vi "B sweep PL.vi"() -> ()   [LabVIEW 2012]
uses:
  <vilib>/Analysis/1siggen.llb/Ramp Pattern by Samples.vi
  <vilib>/Utility/file.llb/Write To Spreadsheet File (DBL).vi
  <vilib>/Analysis/NI_AALBase.lvlib
panel:
  in  "Y Parameters":T1={"Number of Y Steps"=200, "Max Y (V)"=2.0, "Min Y (V)"=-2.0}
  in  "X":T2={"Number of X Steps"=200, "Max X (V)"=2.0, "Min X (V)"=-2.0}
  out "Numeric":dbl
  out "Average intensity (cts/s)":dbl
  in  "file path (dialog if empty)":path
  in  "Time Target (s)":dbl=10.0
  in  "Z Position":dbl
  in  "Y Position":dbl
  in  "X Position":dbl
  in  "Z-track?":bool
  in  "start":dbl format="%0.2f"
  in  "end":dbl=1.0 format="%0.2f"
  in  "samples":i32=128
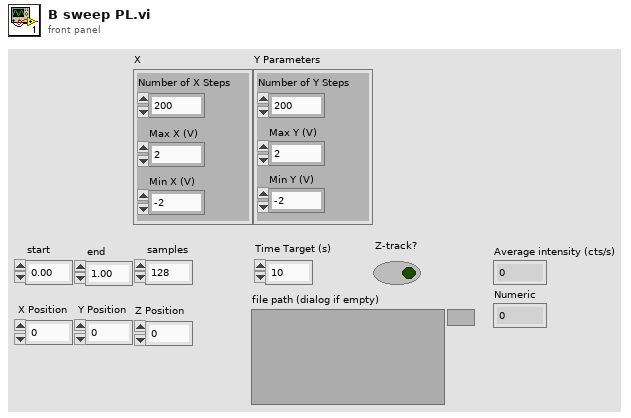
[diagram p1: front panel]
types:
  T1 = cluster{"Number of Y Steps":i32, "Max Y (V)":dbl, "Min Y (V)":dbl}
  T2 = cluster{"Number of X Steps":i32, "Max X (V)":dbl, "Min X (V)":dbl}
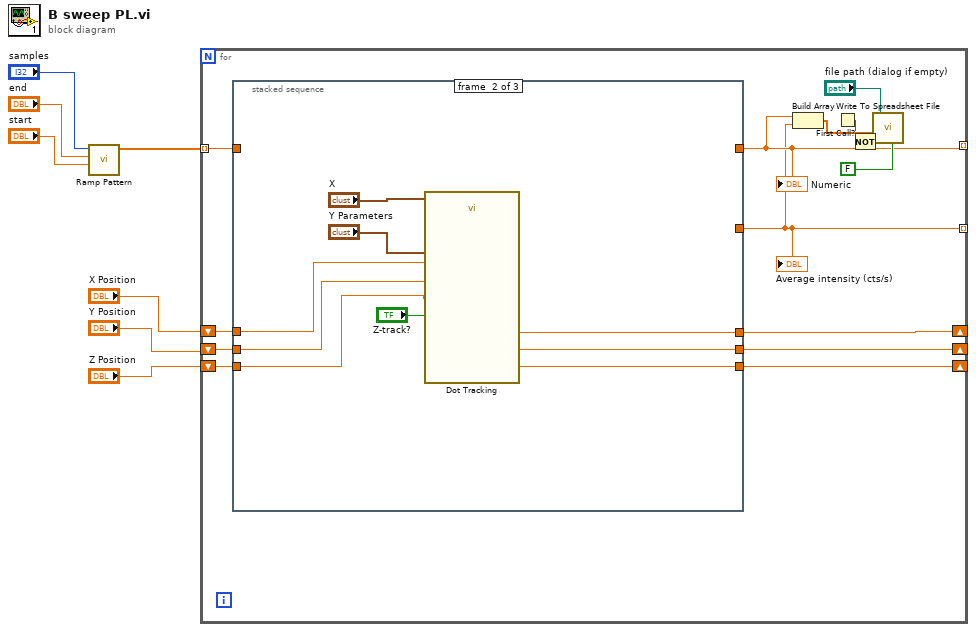
[diagram p0: block diagram]
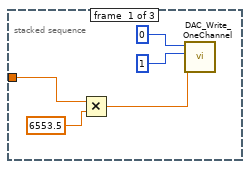
[diagram p2: hidden frame]
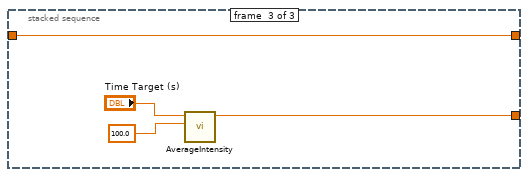
[diagram p3: hidden frame]
diagram:
  n1 = call-poly <vilib>:"Ramp Pattern.vi"("start"="start", "end"="end", "samples"="samples") -> ("Ramp Pattern"=w4:dbl[])  [unwired: 7 in, 1 out]
  n2 = for {
    tunnel: w4 -> [w21] mode=indexing
    shift-right: [w18] -> _
    shift-left: "Z Position" -> [w15]
    shift-right: [w19] -> _
    shift-left: "Y Position" -> [w16]
    shift-right: [w20] -> _
    shift-left: "X Position" -> [w17]
    tunnel: [w11] -> _ mode=indexing
    tunnel: [w12] -> _ mode=indexing
    n3 = stacked-sequence {
      tunnel: w21 -> [w22 _ w36]
      tunnel: [_ w34 _] -> w20
      tunnel: [_ w33 _] -> w19
      tunnel: [_ w32 _] -> w18
      tunnel: w17 -> [_ w31 _]
      tunnel: w16 -> [_ w30 _]
      tunnel: w15 -> [_ w29 _]
      tunnel: [_ _ w37] -> w11
      tunnel: [_ _ w36] -> w12
      frame #0 {
        n4 = Multiply(x=w22, y=6553.5) -> (x*y=w24:dbl)
        n5 = call "DAC_Write_OneChannel.vi"("Value"=w24, "Channel"=u16 1, "DeviceIndex"=u64 0) -> ()  [unwired: 7 in, 2 out]
      }
      frame #1 {
        n6 = call "Dot Tracking.vi"("X"="X", "Y Parameters"="Y Parameters", "X Pos"=w31, "Y pos"=w30, "Z Pos"=w29, "Z-track?"="Z-track?") -> ("X Position"=w34:dbl, "Y Position"=w33:dbl, "Z Position"=w32:dbl)  [unwired: 3 in, 4 out]
      }
      frame #2 {
        n7 = call "AverageIntensity.vi"("rate (Hz)"=100.0, "Time Target (s)"="Time Target (s)") -> ("Average intensity (cts/s)"=w37:dbl)  [unwired: 8 in, 1 out]
      }
    }
    "Average intensity (cts/s)" <- w11
    "Numeric" <- w12
    n8 = Build Array(w12, w11) -> (w10:dbl[])
    n9 = First Call?() -> (First Call?: T/F=w9:bool)
    n10 = Not(x=w9) -> (.not. x?=w8:bool)
    n11 = call-poly <vilib>:"Write To Spreadsheet File.vi"("transpose? (no:F)"=FALSE, "append to file? (new file:F)"=w8, "1D data"=w10, "file path (dialog if empty)"="file path (dialog if empty)") -> ()  [unwired: 4 in, 1 out]
  }
